vi "Import QD Shortcuts.vi"() -> ()   [LabVIEW 2014]
uses:
  <resource>/dialog/lvconfig.llb/LV Config Read String.vi
  <vilib>/Utility/config.llb/Read Key (String).vi
  <vilib>/Utility/config.llb/NI_LVConfig.lvlib
panel:
  in  "QuickDropKeyboardShortcutMappings":bool=TRUE
  in  "QuickDropPanelShortcuts":bool=TRUE
  in  "QuickDropDiagramShortcuts":bool=TRUE
  in  "CustomShortcuts":bool
  in  "System OK Button":bool
  in  "System Cancel Button":bool
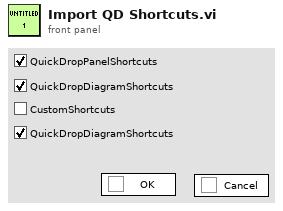
[diagram p1: front panel]
types:
  T1 = typedef "NI_LVConfig.lvlib/Config Data RefNum.ctl" = refnum<k1>
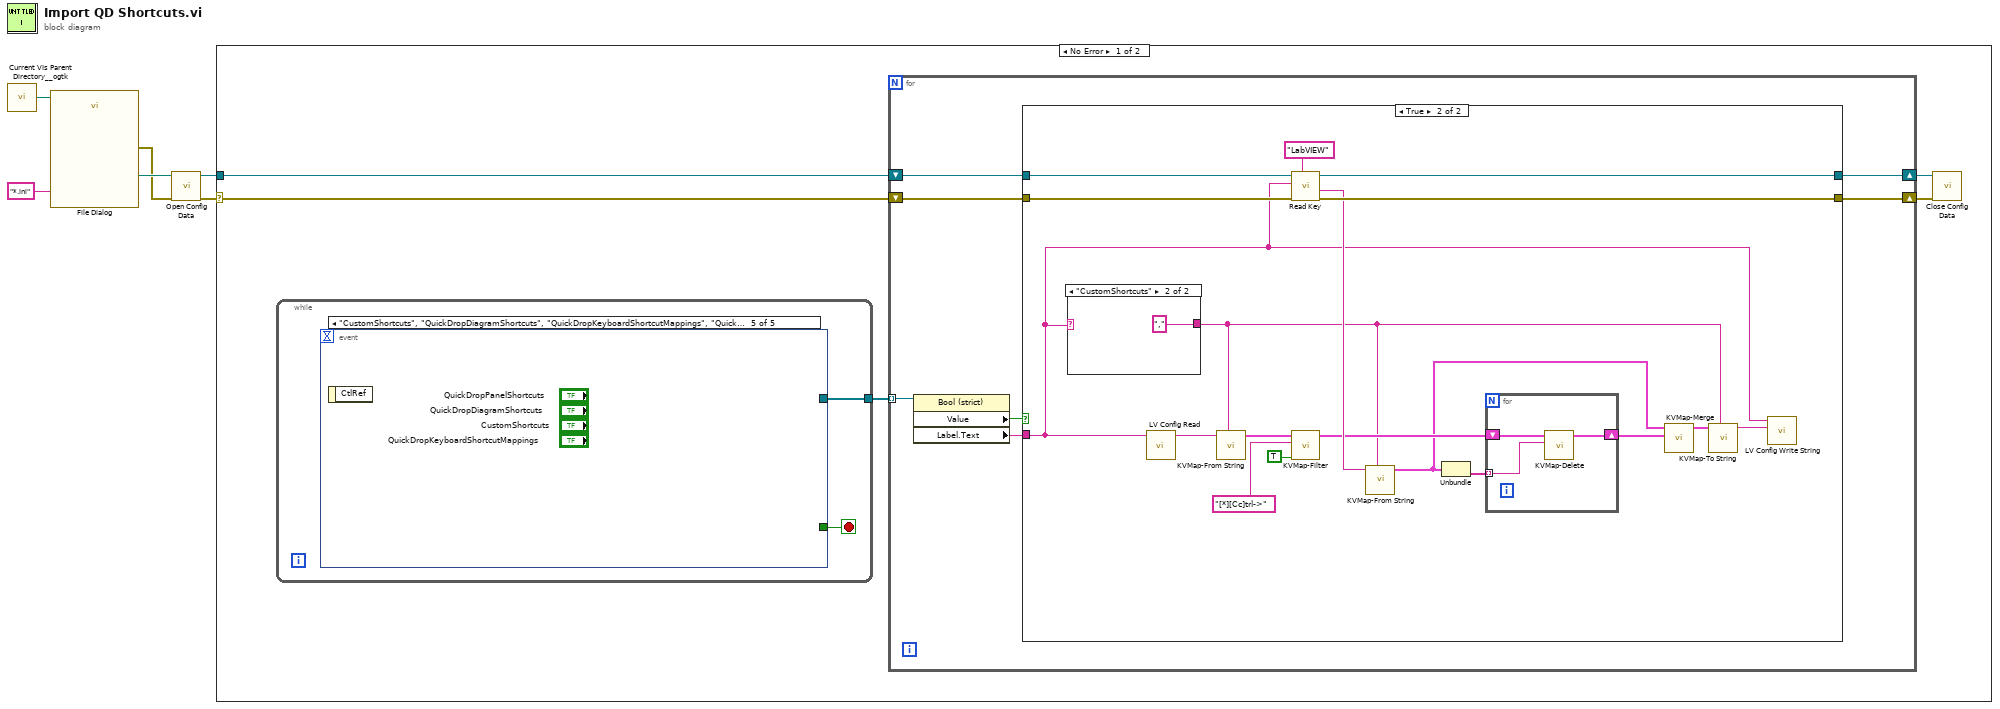
[diagram p0: block diagram]
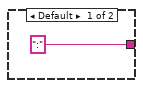
[diagram p3: hidden frame]
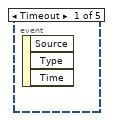
[diagram p4: hidden frame]
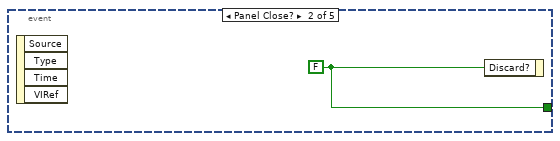
[diagram p5: hidden frame]
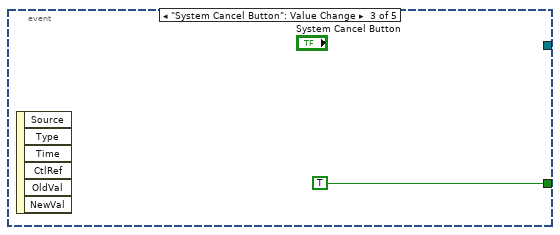
[diagram p6: hidden frame]
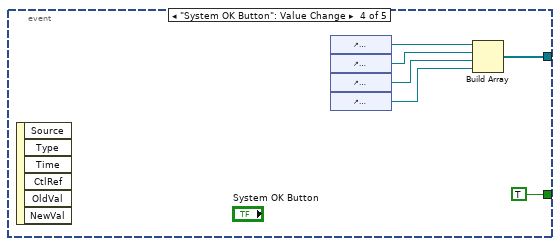
[diagram p7: hidden frame]
diagram:
  n1 = call <userlib>:"Current VIs Parent Directory__ogtk.vi"() -> ("Parent Directory (+ Relative)"=w1:path)  [unwired: 5 in]
  n2 = call "File Dialog"("start path"=w1, "pattern (all files)"="*.ini") -> ("selected path"=w6:path, "error out"=w2:errorcluster)  [unwired: 10 in, 2 out]
  n3 = call <vilib>:"Open Config Data.vi"("error in (no error)"=w2, "configuration file path"=w6) -> ("error out"=w4:errorcluster, "refnum"=w5:T1)  [unwired: 7 in, 1 out]
  n4 = case shown="No Error" w4 {
    selector: w4 -> [w9 _]
    tunnel: w5 -> [w11 _]
    frame No Error {
      n5 = while {
        tunnel: [w44] -> w7
        stop <- w45 stop-if-true
        n6 = event shown="[4] \"CustomShortcuts\", \"QuickDropDiagramShortcuts\", \"QuickDropKeyboardShortcutMappings\", \"QuickDropPanelShortcuts\": Value Change" {
          selector: _ -> [_ _ _ _ _]
          dyn-events: _ -> [_ _ _ _ _]
          timeout: _ -> [_ _ _ _ _]
          tunnel: [_ w46 TRUE ("Discard?") TRUE ("Discard?") _] -> w45
          tunnel: [_ _ _ w52 _] -> w44
          event Timeout {
            n7 = event-data() -> ()  [unwired: 1 in, 3 out]
          }
          event Panel Close? {
            w46 = FALSE ("Discard?")
            n8 = event-data() -> ()  [unwired: 1 in, 4 out]
            n9 = event-data("Discard?"=w46) -> ()  [unwired: 1 in, 1 out]
          }
          event "System Cancel Button": Value Change {
            n10 = event-data() -> ()  [unwired: 1 in, 6 out]
          }
          event "System OK Button": Value Change {
            n11 = event-data() -> ()  [unwired: 1 in, 6 out]
            n12 = control-ref of="QuickDropPanelShortcuts"() -> (w51:refnum<vi>)
            n13 = control-ref of="QuickDropKeyboardShortcutMappings"() -> (w50:refnum<vi>)
            n14 = control-ref of="CustomShortcuts"() -> (w49:refnum<vi>)
            n15 = control-ref of="QuickDropDiagramShortcuts"() -> (w48:refnum<vi>)
            n16 = Build Array(w51, w50, w49, w48) -> (w52:refnum<vi>[])
          }
          event "CustomShortcuts", "QuickDropDiagramShortcuts", "QuickDropKeyboardShortcutMappings", "QuickDropPanelShortcuts": Value Change {
            n17 = event-data() -> ()  [unwired: 1 in, 1 out]
          }
        }
      }
      n18 = for {
        shift-right: [w17] -> w10
        shift-left: w11 -> [w18]
        shift-right: [w15] -> w8
        shift-left: w9 -> [w16]
        tunnel: w7 -> [w14] mode=indexing
        n19 = property class="Bool (strict)"(reference=w14) -> ("Value"=w12:bool, "Label.Text"=w13:string)  [unwired: 1 in, 2 out]
        n20 = case shown="True" w12 {
          tunnel: w18 -> [w20 w34]
          tunnel: [w20 w33] -> w17
          tunnel: w16 -> [w19 w32]
          tunnel: [w19 w31] -> w15
          tunnel: w13 -> [_ w22]
          frame False {
          }
          frame True {
            n21 = case shown="\"CustomShortcuts\"" w22 {
              tunnel: [":" ("delimiter (Tab)") "," ("delimiter (Tab)")] -> w21
              frame Default {
              }
              frame "CustomShortcuts" {
              }
            }
            n22 = call-poly <resource>:"LV Config Read.vi"("key"=w22) -> ("value"=w38:string)  [unwired: 4 in, 2 out]
            n23 = call "KVMap-From String.vi"("delimiter (Tab)"=w21, "value"=w38) -> ("Cluster"=w37:cluster{string[], string[]})  [unwired: 9 in]
            n24 = call-poly <vilib>:"Read Key.vi"("section"="LabVIEW", "error in (no error)"=w32, "key"=w22, "refnum"=w34) -> ("error out"=w31:errorcluster, "value"=w29:string, "refnum out"=w33:T1)  [unwired: 4 in, 1 out]
            n25 = call "KVMap-Filter.vi"("T->First/F->Second(F)"=TRUE, "filter"="[*][Cc]trl->", "Cluster in"=w37) -> ("Cluster out"=w28:cluster{string[], string[]})  [unwired: 8 in]
            n26 = call "KVMap-From String.vi"("delimiter (Tab)"=w21, "value"=w29) -> ("Cluster"=w25:cluster{string[], string[]})  [unwired: 9 in]
            n27 = Unbundle(w25) -> (w27:string[])  [unwired: 1 out]
            n28 = for {
              shift-right: [w42] -> w26
              shift-left: w28 -> [w43]
              tunnel: w27 -> [w41] mode=indexing
              n29 = call "KVMap-Delete.vi"("element"=w41, "Cluster in"=w43) -> ("Cluster out"=w42:cluster{string[], string[]})  [unwired: 9 in]
            }
            n30 = call "KVMap-Merge.vi"("Cluster 2"=w26, "Cluster in"=w25) -> ("Cluster"=w24:cluster{string[], string[]})  [unwired: 8 in]
            n31 = call "KVMap-To String.vi"("string"=w21, "Cluster"=w24) -> ("value"=w23:string)  [unwired: 9 in]
            n32 = call <resource>:"LV Config Write String.vi"("value"=w23, "key"=w22) -> ()  [unwired: 5 in, 1 out]
          }
        }
      }
      n33 = call <vilib>:"Close Config Data.vi"("error in (no error)"=w8, "refnum"=w10) -> ()  [unwired: 8 in, 2 out]
    }
    frame Error {
    }
  }
